vi "Get configuration chain.vi"(8 "error in (no error)":errorcluster, 11 "wavefront sensorBase in":refnum<class "wavefront sensor.lvclass">) -> (0 "error out":errorcluster, 1 "class name":string[](array[string]), 2 "configuration chain":variant[](array[variant]), 3 "wavefront sensorBase out":refnum<class "wavefront sensor.lvclass">)   [LabVIEW 2012, in "wavefront sensor.lvclass"]
doc: "Returns an array of variants containing the configuration clusters of each class in the inheritance chain (lowest child class first), together with an array of all class names in the inheritance chain.\n\nFor classes without configuration cluster, the configuration chain contains empty variants."
uses:
  wavefront sensor.lvclass
  <vilib>/Distrio/Murmex/Murmex/Murmex.lvclass
  wavefront sensor.lvclass/wavefront sensor.ctl
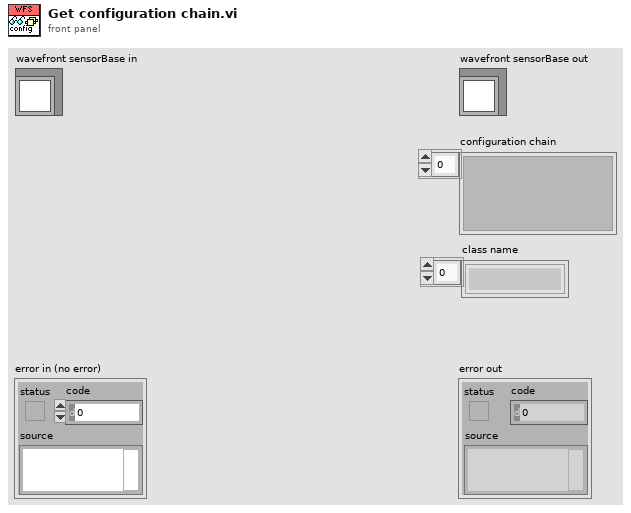
[diagram p1: front panel]
types:
  T1 = typedef "wavefront sensor.lvclass/configuration.ctl" = cluster{"Numeric":dbl}
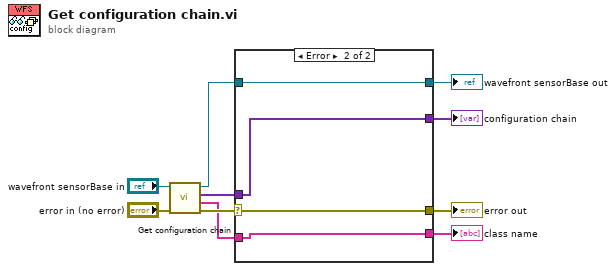
[diagram p0: block diagram]
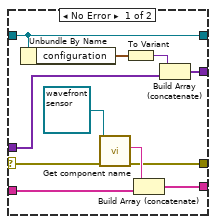
[diagram p2: hidden frame]
diagram:
  n1 = call-parent "Get configuration chain.vi"("error in (no error)"="error in (no error)", "MurmexBase in"="wavefront sensorBase in") -> ("error out"=w8:errorcluster, "class name"=w2:string[], "configuration chain"=w1:variant[], "MurmexBase out"=w6:refnum<class "wavefront sensor.lvclass">)  [unwired: 6 in]
  n2 = case shown="Error" w8 {
    selector: w8 -> [w18 w24]
    tunnel: [w17 w24] -> w7
    tunnel: w6 -> [w15 w25]
    tunnel: [w15 w25] -> w5
    tunnel: [w14 w22] -> w4
    tunnel: [w13 w23] -> w3
    tunnel: w2 -> [w12 w23]
    tunnel: w1 -> [w11 w22]
    frame No Error {
      n3 = Unbundle By Name(w15) -> ("configuration"=w20:T1)
      n4 = call <vilib>:"Get component name.vi"("error in (no error)"=w18, "Murmex in"=refnum<class "wavefront sensor.lvclass"> refnum ("wavefront sensor")) -> ("error out"=w17:errorcluster, "component name"=w19:string)  [unwired: 7 in, 1 out]
      n5 = To Variant(anything=w20) -> (Variant=w21:variant)
      n6 = Build Array (concatenate)(w19, w12) -> (w13:string[])
      n7 = Build Array (concatenate)(w21, w11) -> (w14:variant[])
    }
    frame Error {
    }
  }
  "error out" <- w7
  "wavefront sensorBase out" <- w5
  "configuration chain" <- w4
  "class name" <- w3
